vi "Read Cartesian Lines .vi"(9 "XYGraph in":refnum<class "XYGraph.lvclass">) -> (3 "XYGraph out":refnum<class "XYGraph.lvclass">, 4 "Cartesian Lines":bool)   [LabVIEW 2014, in "Raspberry Pi Compatible Compiler for LabVIEW.lvlib" / "XYGraph.lvclass"]
uses:
  XYGraph.lvclass
  XYGraph.lvclass/XYGraph.ctl
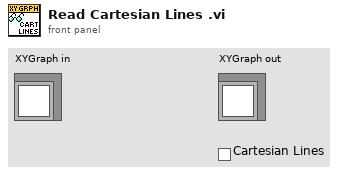
[diagram p1: front panel]
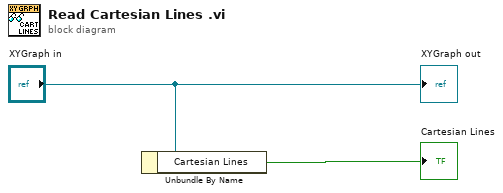
[diagram p0: block diagram]
diagram:
  n1 = Unbundle By Name("XYGraph in") -> ("Cartesian Lines"=→"Cartesian Lines":bool)
  "XYGraph out" <- "XYGraph in"
